vi "Init Input.vi"(8 "actual Values Cluster":T7 {"Cluster"."PumpModeGeneral-Cluster"."dry mode" items=["wet", "dry"]; "Cluster"."PumpModeGeneral-Cluster"."control mode" items=["static", "pid"]; "Cluster"."PumpMode-Cluster"."concentratio mode" items=["water", "reagent"]; "Cluster"."PumpMode-Cluster"."Reagent" items=["HCl", "HF", "NH3", "HG", "PPM", "ORGANIC"]}, 10 "Set Values Cluster (Eingang)":T1(array[cluster]), 11 "Input Cluster (Eingang)":T6 {"PumpModeGeneral-Cluster"."dry mode" items=["wet", "dry"]; "PumpModeGeneral-Cluster"."control mode" items=["static", "pid"]; "PumpMode-Cluster"."concentratio mode" items=["water", "reagent"]; "PumpMode-Cluster"."Reagent" items=["HCl", "HF", "NH3", "HG", "PPM", "ORGANIC"]}) -> (2 "Set Values Cluster (Ausgang)":T1(array[cluster]), 3 "Input Cluster (Ausgang)":T6 {"PumpModeGeneral-Cluster"."dry mode" items=["wet", "dry"]; "PumpModeGeneral-Cluster"."control mode" items=["static", "pid"]; "PumpMode-Cluster"."concentratio mode" items=["water", "reagent"]; "PumpMode-Cluster"."Reagent" items=["HCl", "HF", "NH3", "HG", "PPM", "ORGANIC"]})   [LabVIEW 2020, in "Linearisierung v2.lvlib" / "Gasteiler.lvlib" / "HovaCAL_Interface.lvlib" / "Helper.lvlib"]
uses:
  Helper.lvlib
  Controls/Pump Dry Mode.ctl
  Controls/Pump Control Mode.ctl
  Controls/Pump Concentration Mode.ctl
  Controls/Reagent.ctl
  Controls/Controls.lvlib
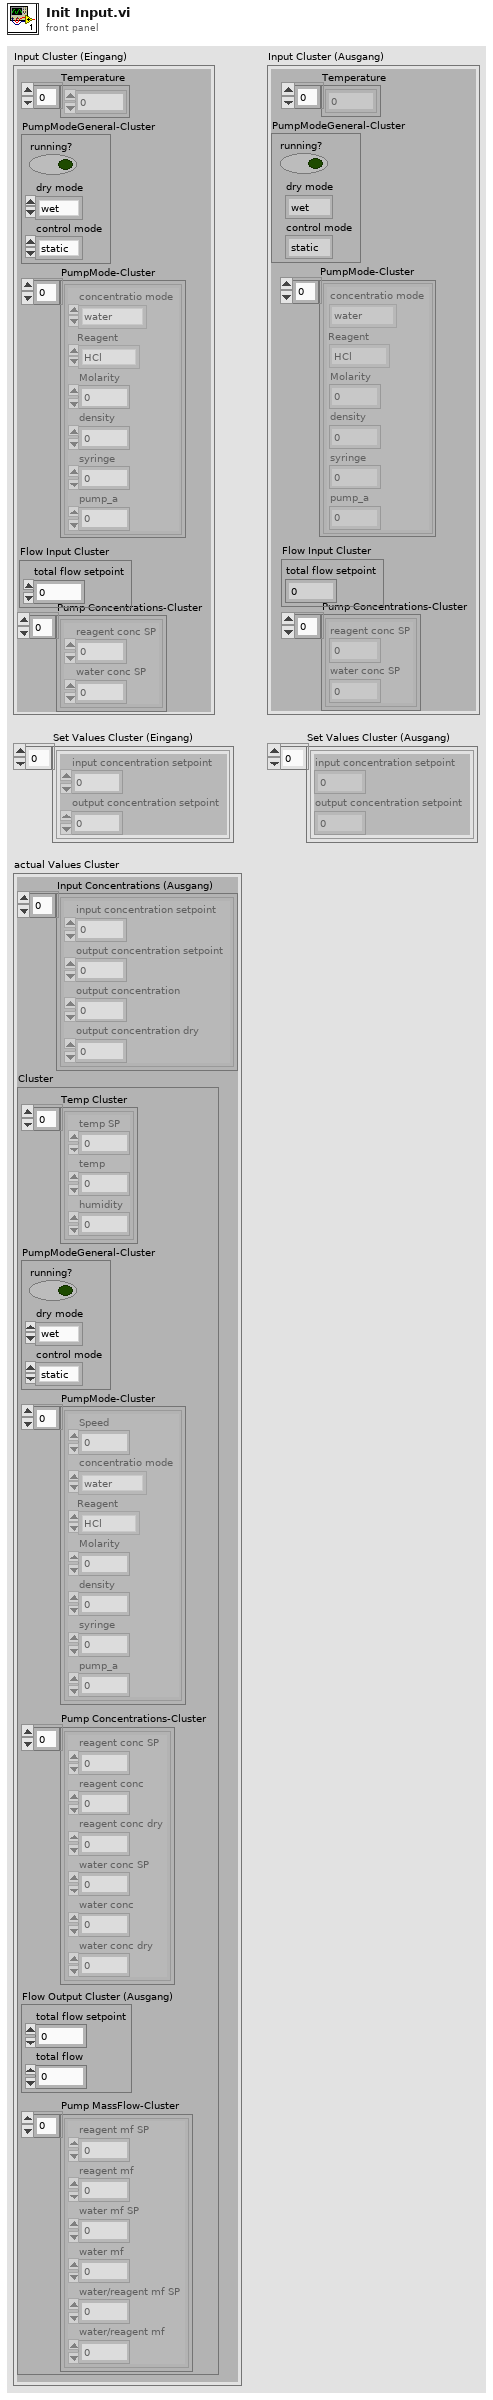
[diagram p1: front panel]
types:
  T1 = cluster{"input concentration setpoint":dbl, "output concentration setpoint":dbl}[]
  T2 = typedef "Linearisierung v2.lvlib/Gasteiler.lvlib/HovaCAL_Interface.lvlib/Controls.lvlib/Pump Dry Mode.ctl" = i32
  T3 = typedef "Linearisierung v2.lvlib/Gasteiler.lvlib/HovaCAL_Interface.lvlib/Controls.lvlib/Pump Control Mode.ctl" = u32
  T4 = typedef "Linearisierung v2.lvlib/Gasteiler.lvlib/HovaCAL_Interface.lvlib/Controls.lvlib/Pump Concentration Mode.ctl" = i32
  T5 = typedef "Linearisierung v2.lvlib/Gasteiler.lvlib/HovaCAL_Interface.lvlib/Controls.lvlib/Reagent.ctl" = i32
  T6 = cluster{"Temperature":dbl[], "PumpModeGeneral-Cluster":cluster{"running?":bool, "dry mode":T2, "control mode":T3}, "PumpMode-Cluster":cluster{"concentratio mode":T4, "Reagent":T5, "Molarity":dbl, "density":dbl, "syringe":dbl, "pump_a":dbl}[], "Flow Input Cluster":cluster{"total flow setpoint":dbl}, "Pump Concentrations-Cluster":cluster{"reagent conc SP":dbl, "water conc SP":dbl}[]}
  T7 = cluster{"Input Concentrations (Ausgang)":cluster{"input concentration setpoint":dbl, "output concentration setpoint":dbl, "output concentration":dbl, "output concentration dry":dbl}[], "Cluster":cluster{"Temp Cluster":cluster{"temp SP":dbl, "temp":dbl, "humidity":dbl}[], "PumpModeGeneral-Cluster":cluster{"running?":bool, "dry mode":T2, "control mode":T3}, "PumpMode-Cluster":cluster{"Speed":dbl, "concentratio mode":T4, "Reagent":T5, "Molarity":dbl, "density":dbl, "syringe":dbl, "pump_a":dbl}[], "Pump Concentrations-Cluster":cluster{"reagent conc SP":dbl, "reagent conc":dbl, "reagent conc dry":dbl, "water conc SP":dbl, "water conc":dbl, "water conc dry":dbl}[], "Flow Output Cluster (Ausgang)":cluster{"total flow setpoint":dbl, "total flow":dbl}, "Pump MassFlow-Cluster":cluster{"reagent mf SP":dbl, "reagent mf":dbl, "water mf SP":dbl, "water mf":dbl, "water/reagent mf SP":dbl, "water/reagent mf":dbl}[]}}
  T8 = cluster{"temp SP":dbl, "temp":dbl, "humidity":dbl}[]
  T9 = cluster{"running?":bool, "dry mode":T2, "control mode":T3}
  T10 = cluster{"Speed":dbl, "concentratio mode":T4, "Reagent":T5, "Molarity":dbl, "density":dbl, "syringe":dbl, "pump_a":dbl}[]
  T11 = cluster{"reagent conc SP":dbl, "reagent conc":dbl, "reagent conc dry":dbl, "water conc SP":dbl, "water conc":dbl, "water conc dry":dbl}[]
  T12 = cluster{"total flow setpoint":dbl, "total flow":dbl}
  T13 = cluster{"reagent mf SP":dbl, "reagent mf":dbl, "water mf SP":dbl, "water mf":dbl, "water/reagent mf SP":dbl, "water/reagent mf":dbl}[]
  T14 = cluster{"input concentration setpoint":dbl, "output concentration setpoint":dbl, "output concentration":dbl, "output concentration dry":dbl}[]
  T15 = cluster{"input concentration setpoint":dbl, "output concentration setpoint":dbl}
  T16 = cluster{"concentratio mode":T4, "Reagent":T5, "Molarity":dbl, "density":dbl, "syringe":dbl, "pump_a":dbl}
  T17 = cluster{"reagent conc SP":dbl, "water conc SP":dbl}
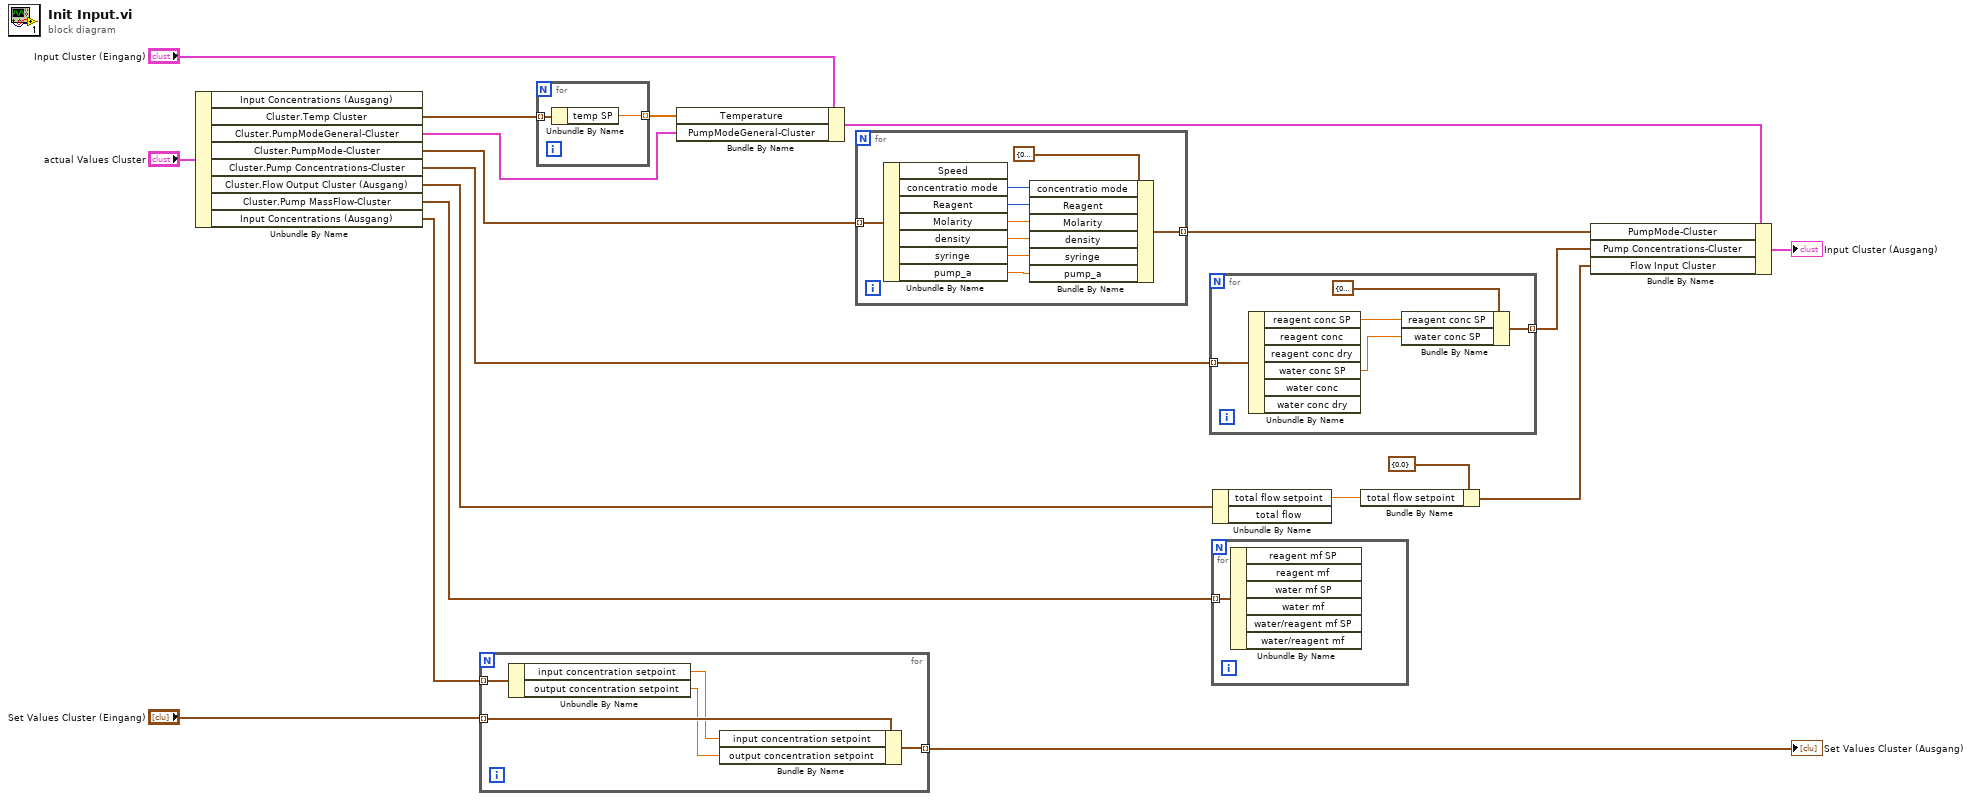
[diagram p0: block diagram]
diagram:
  n1 = Unbundle By Name("actual Values Cluster") -> ("Cluster.Temp Cluster"=w15:T8, "Cluster.PumpModeGeneral-Cluster"=w13:T9, "Cluster.PumpMode-Cluster"=w12:T10, "Cluster.Pump Concentrations-Cluster"=w8:T11, "Cluster.Flow Output Cluster (Ausgang)"=w7:T12, "Cluster.Pump MassFlow-Cluster"=w6:T13, "Input Concentrations (Ausgang)"=w1:T14)  [unwired: 1 out]
  n2 = for {
    tunnel: "Set Values Cluster (Eingang)" -> [w24] mode=indexing
    tunnel: [w23] -> w16 mode=indexing
    tunnel: w1 -> [w22] mode=indexing
    n3 = Unbundle By Name(w22) -> ("input concentration setpoint"=w21:dbl, "output concentration setpoint"=w20:dbl)
    n4 = Bundle By Name(cluster=w24, "input concentration setpoint"=w21, "output concentration setpoint"=w20) -> (w23:T15)
  }
  "Set Values Cluster (Ausgang)" <- w16
  n5 = for {
    tunnel: w15 -> [w26] mode=indexing
    tunnel: [w25] -> w14 mode=indexing
    n6 = Unbundle By Name(w26) -> ("temp SP"=w25:dbl)
  }
  n7 = Bundle By Name(cluster="Input Cluster (Eingang)", "Temperature"=w14, "PumpModeGeneral-Cluster"=w13) -> (w11:T6)
  n8 = for {
    tunnel: w12 -> [w35] mode=indexing
    tunnel: [w28] -> w10 mode=indexing
    n9 = Unbundle By Name(w35) -> ("concentratio mode"=w34:T4, "Reagent"=w33:T5, "Molarity"=w32:dbl, "density"=w31:dbl, "syringe"=w30:dbl, "pump_a"=w27:dbl)  [unwired: 1 out]
    n10 = Bundle By Name(cluster=T16 {"concentratio mode"=0, "Reagent"=0, "Molarity"=0.0, "density"=0.0, "syringe"=0.0, "pump_a"=0.0} ("PumpMode-Cluster"), "concentratio mode"=w34, "Reagent"=w33, "Molarity"=w32, "density"=w31, "syringe"=w30, "pump_a"=w27) -> (w28:T16)
  }
  n11 = for {
    tunnel: w8 -> [w40] mode=indexing
    tunnel: [w36] -> w5 mode=indexing
    n12 = Unbundle By Name(w40) -> ("reagent conc SP"=w38:dbl, "water conc SP"=w37:dbl)  [unwired: 4 out]
    n13 = Bundle By Name(cluster=T17 {"reagent conc SP"=0.0, "water conc SP"=0.0} ("Ausgangs-Cluster"), "reagent conc SP"=w38, "water conc SP"=w37) -> (w36:T17)
  }
  n14 = for {
    tunnel: w6 -> [w41] mode=indexing
    n15 = Unbundle By Name(w41) -> ()  [unwired: 6 out]
  }
  n16 = Unbundle By Name(w7) -> ("total flow setpoint"=w2:dbl)  [unwired: 1 out]
  n17 = Bundle By Name(cluster=cluster{"total flow setpoint":dbl} {"total flow setpoint"=0.0} ("Flow Input Cluster"), "total flow setpoint"=w2) -> (w4:cluster{"total flow setpoint":dbl})
  n18 = Bundle By Name(cluster=w11, "PumpMode-Cluster"=w10, "Pump Concentrations-Cluster"=w5, "Flow Input Cluster"=w4) -> (→"Input Cluster (Ausgang)":T6)
